vi "Main.vi"(8 "error in":errorcluster, 11 "Timer in":refnum<class "Timer.lvclass">) -> (0 "error out":errorcluster, 3 "Timer out":refnum<class "Timer.lvclass">)   [LabVIEW 2022 SP3, in "Timer.lvclass"]
doc: "The Queued Message Handler of a Worker."
uses:
  Timer.lvclass
  C:/Program Files (x86)/National Instruments/LabVIEW 2022/vi.lib/addons/_Workers/Library/Classes/Worker/Worker.lvclass
  Timer.lvclass/Timer.ctl
  <vilib>/addons/_Workers/Library/Classes/Message Queue/Message Queue.lvclass
  <vilib>/addons/_Workers/Library/Case Label.ctl
  <vilib>/addons/_Workers/Library/Classes/Worker/Worker.lvclass/Worker.ctl
  <vilib>/addons/_Workers/Library/Classes/Message/Enqueue Message to Self v2.vi
  <vilib>/addons/_Workers/Library/Classes/Message/Enqueue Message to Self v2 - Silent Mode.vi
  <vilib>/addons/_Workers/Library/Classes/Message/Enqueue Message to Queue.vi
  Initialization Data.ctl
  <vilib>/addons/_Workers/Library/Classes/Message/Message.lvclass
  <vilib>/addons/_Workers/Library/Workers.lvlib
  <vilib>/addons/_Workers/Library/Classes/Worker/Worker.lvclass
  C:/Program Files (x86)/National Instruments/LabVIEW 2022/vi.lib/addons/_Workers/Library/Classes/Workers Object/Workers Object.lvclass
  C:/Users/chrismadlax/Desktop/LVSampleCode/ArduinoController/Workers/Timer/Timer.lvclass
panel:
  out "x-y":dbl
  out "CurrentTime":timestamp
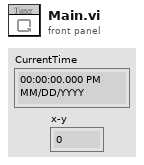
[diagram p1: front panel]
types:
  T1 = typedef "Timer.lvclass/Initialization Data.ctl" = cluster{"String":string}
  T2 = typedef "Workers.lvlib/Case Label.ctl" = string
  T3 = cluster{"MessageQ":refnum<class "Message Queue.lvclass">, "CaseLabel":T2}
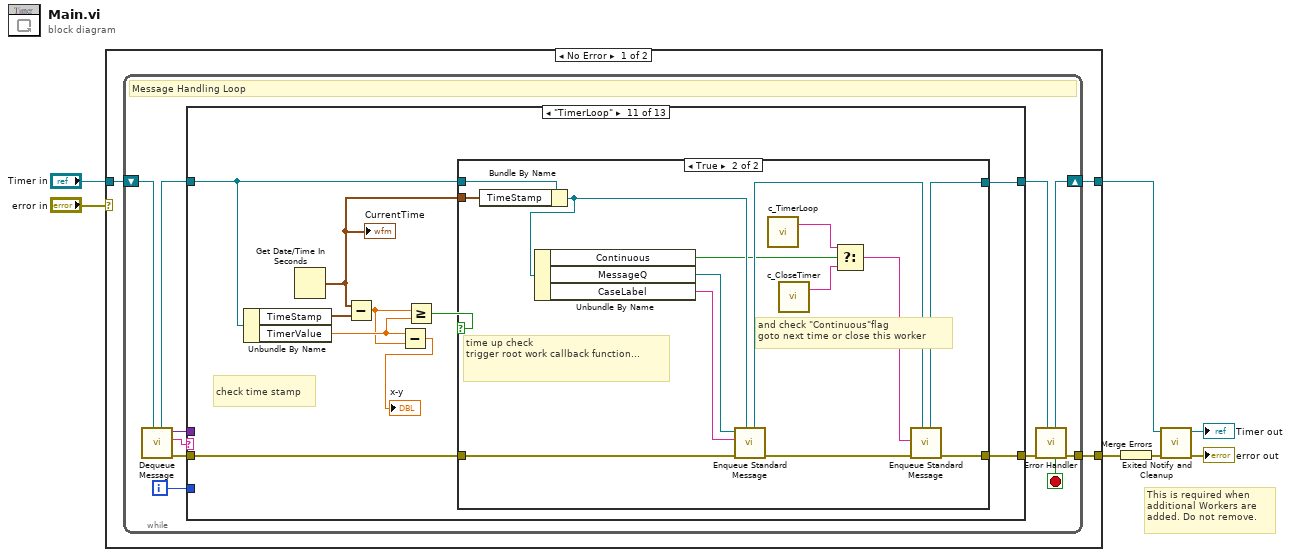
[diagram p0: block diagram]
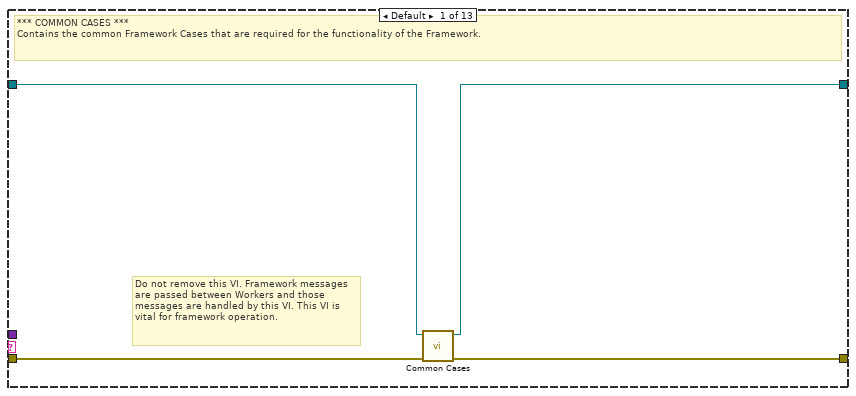
[diagram p2: hidden frame]
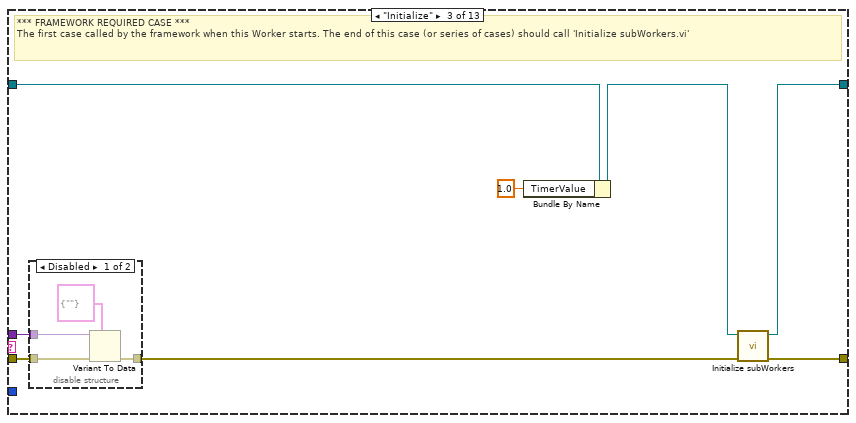
[diagram p4: hidden frame]
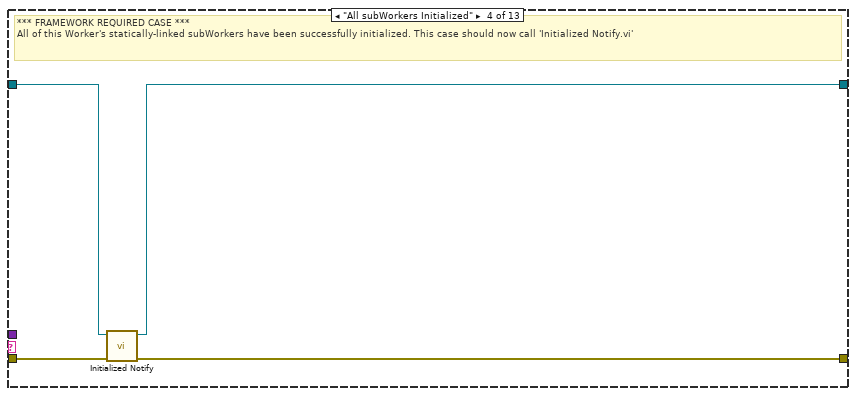
[diagram p6: hidden frame]
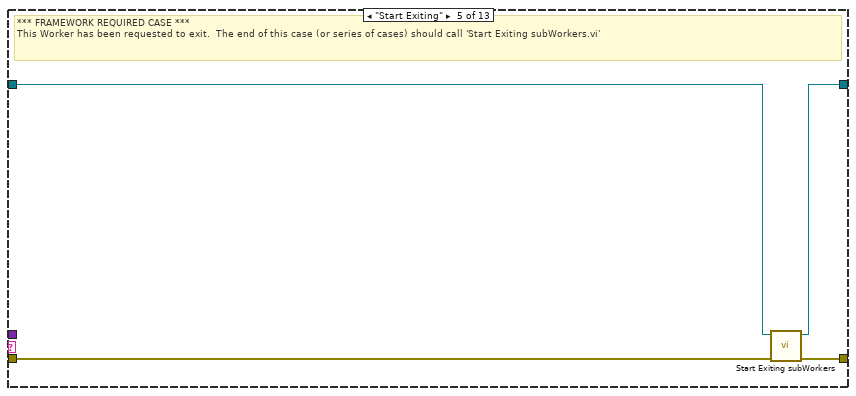
[diagram p7: hidden frame]
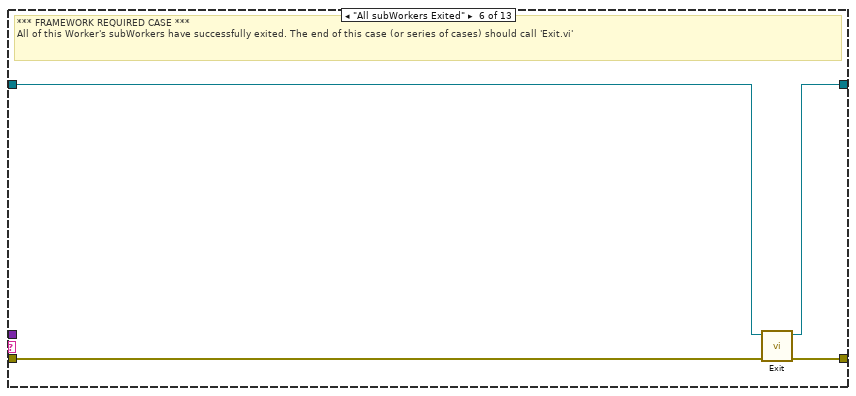
[diagram p8: hidden frame]
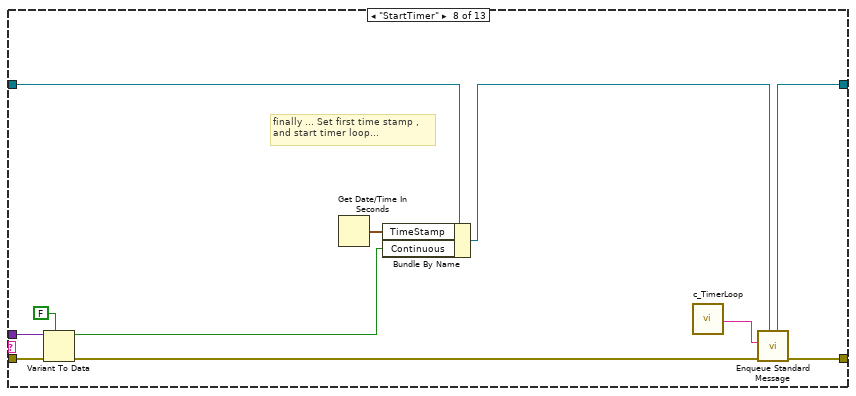
[diagram p10: hidden frame]
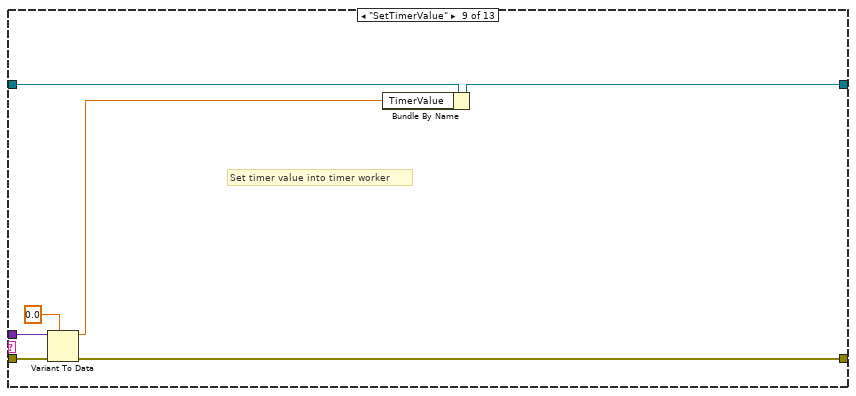
[diagram p11: hidden frame]
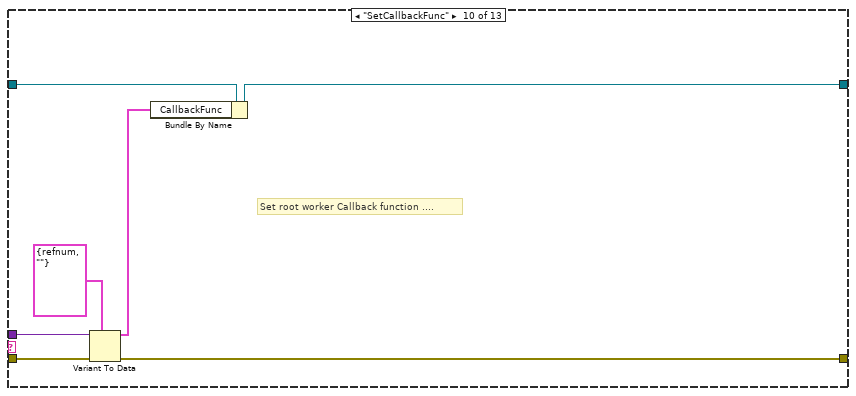
[diagram p12: hidden frame]
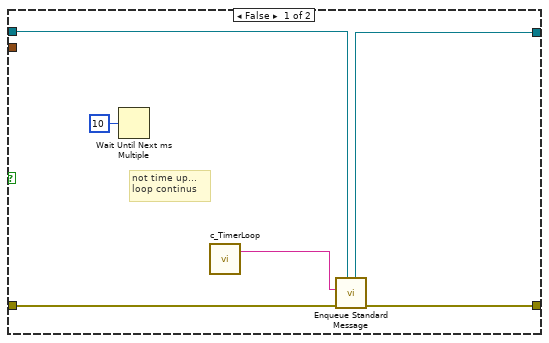
[diagram p13: hidden frame]
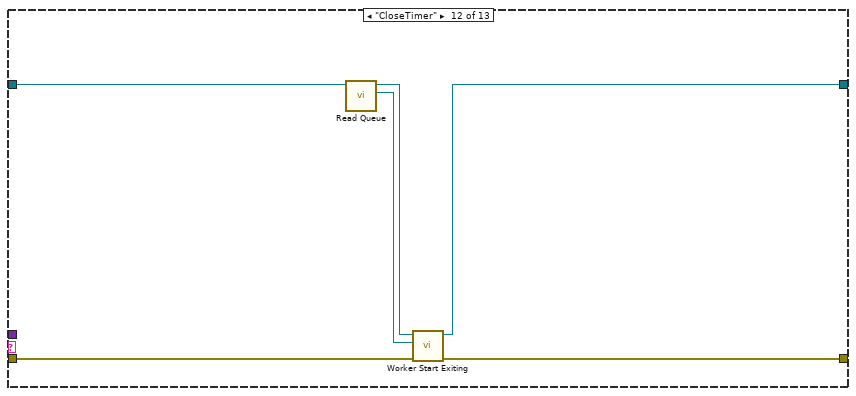
[diagram p14: hidden frame]
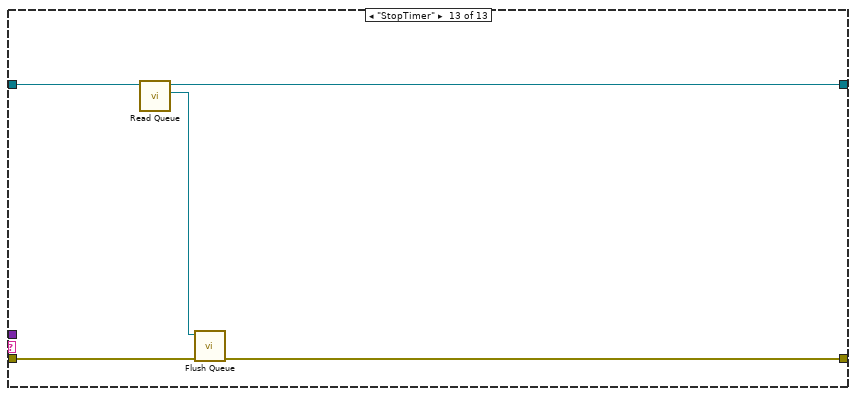
[diagram p15: hidden frame]
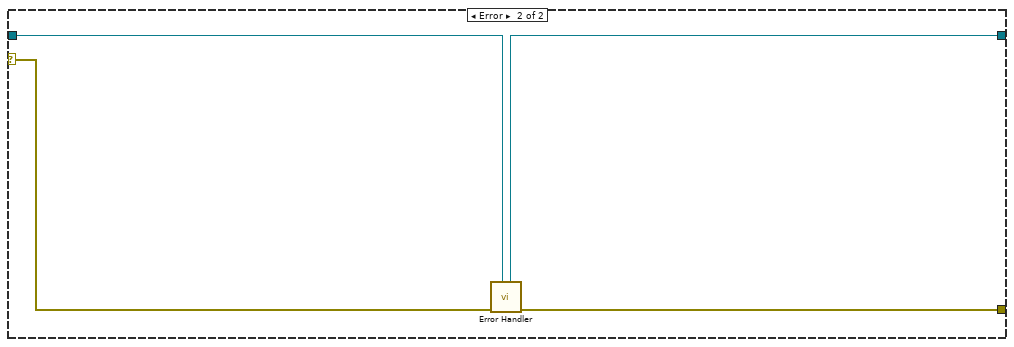
[diagram p16: hidden frame]
diagram:
  # "This is required when additional Workers are added. Do not remove."
  n1 = case shown="No Error" "error in" {
    tunnel: "Timer in" -> [w8 w122]
    tunnel: [w10 w123] -> w6
    tunnel: [w9 w121] -> w7
    selector: "error in" -> [_ w124]
    frame No Error {
      n2 = while {
        shift-right: [w19] -> w9
        shift-left: w8 -> [w21]
        tunnel: [w20] -> w10
        i -> [w11]
        stop <- w12 stop-if-true
        # "Message Handling Loop"
        n3 = call-dynamic "Dequeue Message.vi"("Worker"=w21) -> ("error out"=w18:errorcluster, "Case out"=w13:string, "Data out"=w14:variant, "Worker out"=w16:refnum<class "Timer.lvclass">)  [unwired: 6 in, 1 out]
        n4 = case "Worker MHL Case Structure (DO NOT CHANGE LABEL NAME)" shown="\"TimerLoop\"" w13 {
          tunnel: w18 -> [w25 w26 w33 w44 w45 w52 w53 w59 w72 w79 w89 w115 w120]
          tunnel: [w24 w26 w35 w43 w48 w51 w53 w63 w69 w77 w87 w114 w117] -> w17
          tunnel: w16 -> [w23 w27 w32 w42 w46 w50 w54 w65 w71 w78 w85 w113 w119]
          tunnel: [w22 w27 w34 w41 w47 w49 w54 w61 w70 w74 w86 w112 w118] -> w15
          tunnel: w14 -> [_ _ w30 _ _ _ _ w57 w68 w76 _ _ _]
          tunnel: w11 -> [_ _ _ _ _ _ _ _ _ _ _ _ _]
          frame Default {
            # "Do not remove this VI. Framework messages are passed between Workers and those messages are handled by this VI. This VI is vital for framework operation."
            # "*** COMMON CASES ***\nContains the common Framework Cases that are required for the functionality of the Framework."
            n5 = call-dynamic "Common Cases.vi"("error in"=w25, "Worker in"=w23) -> ("error out"=w24:errorcluster, "Worker out"=w22:refnum<class "Timer.lvclass">)  [unwired: 8 in]
          }
          frame "------ FRAMEWORK REQUIRED CASES ------" {
            # "Start of Framework Required Cases"
          }
          frame "Initialize" {
            # "*** FRAMEWORK REQUIRED CASE ***\nThe first case called by the framework when this Worker starts. The end of this case (or series of cases) should call 'Initialize subWorkers.vi'"
            n6 = disable-structure shown="Disabled" {
              disable-tunnel: w33 -> [w39 w40]
              disable-tunnel: [w38 w40] -> w31
              disable-tunnel: w30 -> [w36 _]
              frame Disabled {
                n7 = Variant To Data(error in=w39, type=T1 {"String"=""} ("Cluster"), Variant=w36) -> (error out=w38:errorcluster)  [unwired: 1 out]
              }
              frame Enabled {
              }
            }
            n8 = Bundle By Name(cluster=w32, "TimerValue"=1.0) -> (w29:refnum<class "Timer.lvclass">)
            n9 = call-dynamic "Initialize subWorkers.vi"("error in"=w31, "Worker"=w29) -> ("error out"=w35:errorcluster, "dup Worker out"=w34:refnum<class "Timer.lvclass">)  [unwired: 8 in]
          }
          frame "All subWorkers Initialized" {
            # "*** FRAMEWORK REQUIRED CASE ***\nAll of this Worker's statically-linked subWorkers have been successfully initialized. This case should now call 'Initialized Notify.vi'"
            n10 = call-dynamic "Initialized Notify.vi"("error in"=w44, "Worker"=w42) -> ("error out"=w43:errorcluster, "dup Worker out"=w41:refnum<class "Timer.lvclass">)  [unwired: 8 in]
          }
          frame "Start Exiting" {
            # "*** FRAMEWORK REQUIRED CASE ***\nThis Worker has been requested to exit.  The end of this case (or series of cases) should call 'Start Exiting subWorkers.vi'"
            n11 = call-dynamic "Start Exiting subWorkers.vi"("error_in"=w45, "Worker"=w46) -> ("error out"=w48:errorcluster, "dup Worker out"=w47:refnum<class "Timer.lvclass">)  [unwired: 8 in]
          }
          frame "All subWorkers Exited" {
            # "*** FRAMEWORK REQUIRED CASE ***\nAll of this Worker's subWorkers have successfully exited. The end of this case (or series of cases) should call 'Exit.vi'"
            n12 = call-dynamic "Exit.vi"("error_in"=w52, "Worker"=w50) -> ("error out"=w51:errorcluster, "dup Worker out"=w49:refnum<class "Timer.lvclass">)  [unwired: 8 in]
          }
          frame "-----------------------------------------------" {
            # "End of Framework Required Cases"
          }
          frame "StartTimer" {
            # "finally ... Set first time stamp ,\nand start timer loop..."
            n13 = Variant To Data(error in=w59, type=FALSE, Variant=w57) -> (data=w55:bool, error out=w58:errorcluster)
            n14 = Get Date/Time In Seconds() -> (seconds since 1Jan1904=w64:timestamp)
            n15 = Bundle By Name(cluster=w65, "TimeStamp"=w64, "Continuous"=w55) -> (w62:refnum<class "Timer.lvclass">)
            n16 = call "c_TimerLoop.vi"() -> ("Case Label"=w60:T2)  [unwired: 1 in]
            n17 = call-poly <vilib>:"Enqueue Standard Message.vi"("Worker"=w62, "error in"=w58, "Case Label"=w60) -> ("error out"=w63:errorcluster, "dup Worker out"=w61:refnum<class "Timer.lvclass">)  [unwired: 7 in]
          }
          frame "SetTimerValue" {
            # "Set timer value into timer worker"
            n18 = Variant To Data(error in=w72, type=0.0, Variant=w68) -> (data=w66:dbl, error out=w69:errorcluster)
            n19 = Bundle By Name(cluster=w71, "TimerValue"=w66) -> (w70:refnum<class "Timer.lvclass">)
          }
          frame "SetCallbackFunc" {
            # "Set root worker Callback function ...."
            n20 = Variant To Data(error in=w79, type=T3 {"MessageQ"=refnum, "CaseLabel"=""} ("cluster"), Variant=w76) -> (data=w73:T3, error out=w77:errorcluster)
            n21 = Bundle By Name(cluster=w78, "CallbackFunc"=w73) -> (w74:refnum<class "Timer.lvclass">)
          }
          frame "TimerLoop" {
            # "check time stamp"
            n22 = Unbundle By Name(w85) -> ("TimeStamp"=w88:timestamp, "TimerValue"=w82:dbl)
            n23 = Get Date/Time In Seconds() -> (seconds since 1Jan1904=w83:timestamp)
            "CurrentTime" <- w83
            n24 = Subtract(x=w83, y=w88) -> (x-y=w81:dbl)
            n25 = Subtract(x=w82, y=w81) -> (x-y=→"x-y":dbl)
            n26 = Greater Or Equal?(x=w81, y=w82) -> (x >= y?=w84:bool)
            n27 = case shown="True" w84 {
              tunnel: w89 -> [w95 w109]
              tunnel: [w93 w102] -> w87
              tunnel: [w91 w100] -> w86
              tunnel: w85 -> [w92 w107]
              tunnel: w83 -> [_ w106]
              frame False {
                # "not time up...\nloop continus"
                n28 = Wait Until Next ms Multiple(millisecond multiple=u32 10) -> ()  [unwired: 1 out]
                n29 = call "c_TimerLoop.vi"() -> ("Case Label"=w90:T2)  [unwired: 1 in]
                n30 = call-poly <vilib>:"Enqueue Standard Message.vi"("Worker"=w92, "error in"=w95, "Case Label"=w90) -> ("error out"=w93:errorcluster, "dup Worker out"=w91:refnum<class "Timer.lvclass">)  [unwired: 7 in]
              }
              frame True {
                # "and check \"Continuous\"flag \ngoto next time or close this worker"
                # "time up check\ntrigger root work callback function..."
                n31 = Bundle By Name(cluster=w107, "TimeStamp"=w106) -> (w105:refnum<class "Timer.lvclass">)
                n32 = Unbundle By Name(w105) -> ("Continuous"=w99:bool, "MessageQ"=w104:refnum<class "Message Queue.lvclass">, "CaseLabel"=w103:T2)
                n33 = call-poly <vilib>:"Enqueue Standard Message.vi"("Worker"=w105, "error in"=w109, "Case Label"=w103, "Message Queue"=w104) -> ("error out"=w108:errorcluster, "dup Worker out"=w101:refnum<class "Timer.lvclass">)  [unwired: 5 in, 1 out]
                n34 = call "c_TimerLoop.vi"() -> ("Case Label"=w98:T2)  [unwired: 1 in]
                n35 = call "c_CloseTimer.vi"() -> ("Case Label"=w96:T2)  [unwired: 1 in]
                n36 = Select(t=w98, s=w99, f=w96) -> (s? t:f=w97:T2)
                n37 = call-poly <vilib>:"Enqueue Standard Message.vi"("Worker"=w101, "error in"=w108, "Case Label"=w97) -> ("error out"=w102:errorcluster, "dup Worker out"=w100:refnum<class "Timer.lvclass">)  [unwired: 7 in]
              }
            }
          }
          frame "CloseTimer" {
            n38 = call <vilib>:"Read Queue.vi"("Worker"=w113) -> ("Message Queue out"=w110:refnum<class "Message Queue.lvclass">, "dup Worker out"=w111:refnum<class "Timer.lvclass">)  [unwired: 9 in]
            n39 = call-dynamic "Worker Start Exiting.vi"("error_in"=w115, "Message Queue"=w110, "Worker"=w111) -> ("error out"=w114:errorcluster, "dup Worker out"=w112:refnum<class "Timer.lvclass">)  [unwired: 7 in]
          }
          frame "StopTimer" {
            n40 = call <vilib>:"Read Queue.vi"("Worker"=w119) -> ("Message Queue out"=w116:refnum<class "Message Queue.lvclass">, "dup Worker out"=w118:refnum<class "Timer.lvclass">)  [unwired: 9 in]
            n41 = call <vilib>:"Flush Queue.vi"("error in (no error)"=w120, "Message Queue"=w116) -> ("error out"=w117:errorcluster)  [unwired: 7 in, 2 out]
          }
        }
        n42 = call-dynamic "Error Handler.vi"("Worker"=w15, "error_in"=w17) -> ("error out"=w20:errorcluster, "Stop Loop"=w12:bool, "Worker out"=w19:refnum<class "Timer.lvclass">)  [unwired: 7 in]
      }
    }
    frame Error {
      n43 = call-dynamic "Error Handler.vi"("Worker"=w122, "error_in"=w124) -> ("error out"=w123:errorcluster, "Worker out"=w121:refnum<class "Timer.lvclass">)  [unwired: 7 in, 1 out]
    }
  }
  n44 = Merge Errors(w6) -> (w3:errorcluster)
  n45 = call-dynamic "Exited Notify and Cleanup.vi"("error_in"=w3, "Worker"=w7) -> ("error out"=→"error out":errorcluster, "dup Worker out"=→"Timer out":refnum<class "Timer.lvclass">)  [unwired: 8 in]
